vi "写入服务器信息.vi"(8 "error in (no error)":errorcluster caption="错误输入（无错误）", 10 "服务器信息":cluster{"host":string, "port":u16}={"host"="121.36.219.111", "port"=10001}, 11 "TCP_client输入":refnum<class "TCP_client.lvclass">) -> (0 "error out":errorcluster caption="错误输出", 3 "TCP_client输出":refnum<class "TCP_client.lvclass">)   [LabVIEW 2016, in "数据传输系统-06.lvlib" / "update.lvlib" / "TCP_client.lvclass"]
uses:
  TCP_client.lvclass
  TCP_client.lvclass/TCP_client.ctl
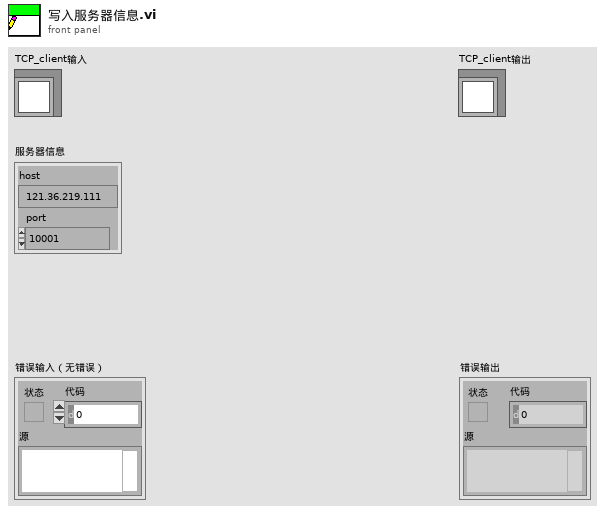
[diagram p1: front panel]
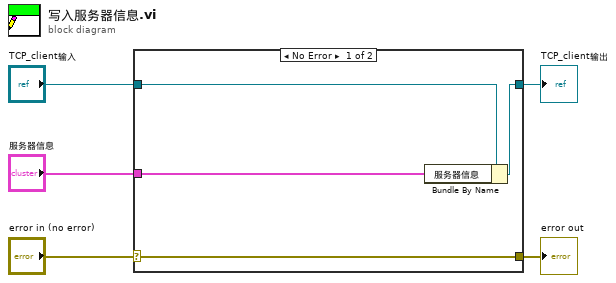
[diagram p0: block diagram]
diagram:
  n1 = case shown="No Error" "error in (no error)" {
    selector: "error in (no error)" -> [w9 w10]
    tunnel: [w9 w10] -> w4
    tunnel: [w7 w11] -> w2
    tunnel: "TCP_client输入" -> [w8 w11]
    tunnel: "服务器信息" -> [w6 _]
    frame No Error {
      n2 = Bundle By Name(cluster=w8, "服务器信息"=w6) -> (w7:refnum<class "TCP_client.lvclass">)
    }
    frame Error {
    }
  }
  "error out" <- w4
  "TCP_client输出" <- w2
